vi "Register Main UI Events.vi"(8 "error in (no error)":errorcluster, 11 "GVIWebProcessorApp in":refnum<class "GVIWebProcessorApp.lvclass">) -> (0 "error out":errorcluster, 2 "Main UI Event Reg":refnum<event-registration>, 3 "GVIWebProcessorApp out":refnum<class "GVIWebProcessorApp.lvclass">)   [LabVIEW 2020, in "PicoG-Processor.lvlib" / "GVIWebProcessorApp.lvclass"]
uses:
  GVIWebProcessorApp.lvclass
  Refresh Event Data.ctl
  Close Event Data.ctl
  Set Collapsed UI Event.ctl
  WebProjectWatcher/Web Build.ctl
  WebProjectWatcher/WebProjectWatcher.lvclass
  Main Events.ctl
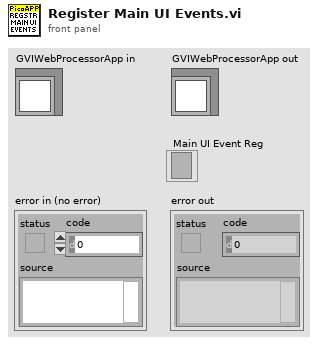
[diagram p1: front panel]
types:
  T1 = typedef "PicoG-Processor.lvlib/GVIWebProcessorApp.lvclass/Main Events.ctl" = cluster{"Refresh":refnum<user-event>, "Close":refnum<user-event>, "Set Collapse":refnum<user-event>, "Builds":refnum<user-event>, "Deploy":refnum<user-event>}
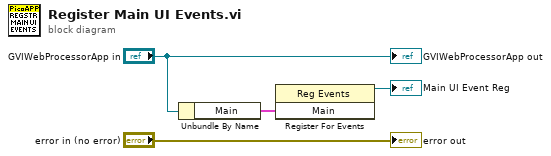
[diagram p0: block diagram]
diagram:
  n1 = Unbundle By Name("GVIWebProcessorApp in") -> ("Main"=w3:T1)
  n2 = register-events(w3) -> (reference out=→"Main UI Event Reg":refnum<event-registration>)  [unwired: 2 in, 1 out]
  "error out" <- "error in (no error)"
  "GVIWebProcessorApp out" <- "GVIWebProcessorApp in"
